vi "NF90 calibrator.vi"(9 "Ports":T1, 10 "channel index":i8, 11 "data server address":string="calcium") -> ()   [LabVIEW 2012]
doc: "Illustrates the simplest form of TCP data acquisition using a TCP data server.\n\n\nCreated by Monroe Weber-Shirk\nCornell University\nmw24@cornell.edu\nJanuary 2000"
uses:
  NF90 move.ctl
  Axis.ctl
  DAC apps/support/method.ctl
  DataServer/command cluster.ctl
  DataServer/command.ctl
  DAQ configuration/Sensor array.ctl
  DAQ configuration/channel identifier.ctl
  NF90 commands.ctl
  calibration/global scale array.vi
  DataServer/Server Stats.vi
panel:
  in  "Go to Start":bool
  in  "Save Data":bool
  in  "Save Calibration":bool
  in  "Calibrate":bool
  in  "Go Home":bool
  in  "Done":bool
  in  "Find Home":bool
  in  "Acceleration":u8=6 min=1 max=50 step=1
  in  "Speed":sgl=1.0 min=0 max=3 format="%.3f"
  out "sample time":dbl format="%.2f"
  out "Sample rate":dbl format="%.2f"
  out "Error":cluster{sgl[], dbl[]}[](graph)
  in  "polynomial order":i32=2 min=1 max=5 step=1
  out "Calibation data":cluster{sgl[], "Best Polynomial Fit":dbl[]}[](graph)
  in  "Number of locations":u8=5 min=2 step=1
  in  "Start position":sgl min=-1048575 max=1048575 format="%.2f"
  in  "delay after move":u32=1000
  in  "Final position":sgl=10.0 min=-1048575 max=1048575 format="%.2f"
  in  "data points to acquire":u32=1000 min=1
  in  "Scans per Sample":i32=1 min=1
  in  "Connection ID":refnum<k5>
  in  "method":T3={"sampling interval"=0.1, "samples to average"=1, "data interval"=0.0, "stream data"=FALSE, "file path"=refnum, "command"={"command"=enum."Idle", "start time (ms)"=0, "Channel Indices"=[], "Scans per Sample"=1}} {"command"."Scans per Sample" min=1; "data interval" format="%.2f"; "samples to average" min=1 step=1; "sampling interval" format="%.2f"}
  in  "move":T6={"axis"=enum."Z", "Increment"=0.0, "Speed"=1.0, "Acceleration"=1} {"Speed" min=0 format="%.3f"; "Acceleration" min=1 max=50 step=1; "Increment" format="%.3f"}
  in  "Home offset from limit switch":sgl min=-1048575 max=1048575 format="%.2f"
  out "Position":sgl(slide) min=0 max=6 step=-1 scale=0.0..1.0 scale format="%.2f"
  in  "serial port":refnum<visa-resource-name>="COM1"
  in  "stop":bool
  # "cm"
  # "cm/s"
  # "cm/s^2"
  # "cm"
  # "cm"
  # "Hz"
  # "s"
  # "ms"
  # "s"
  # "s"
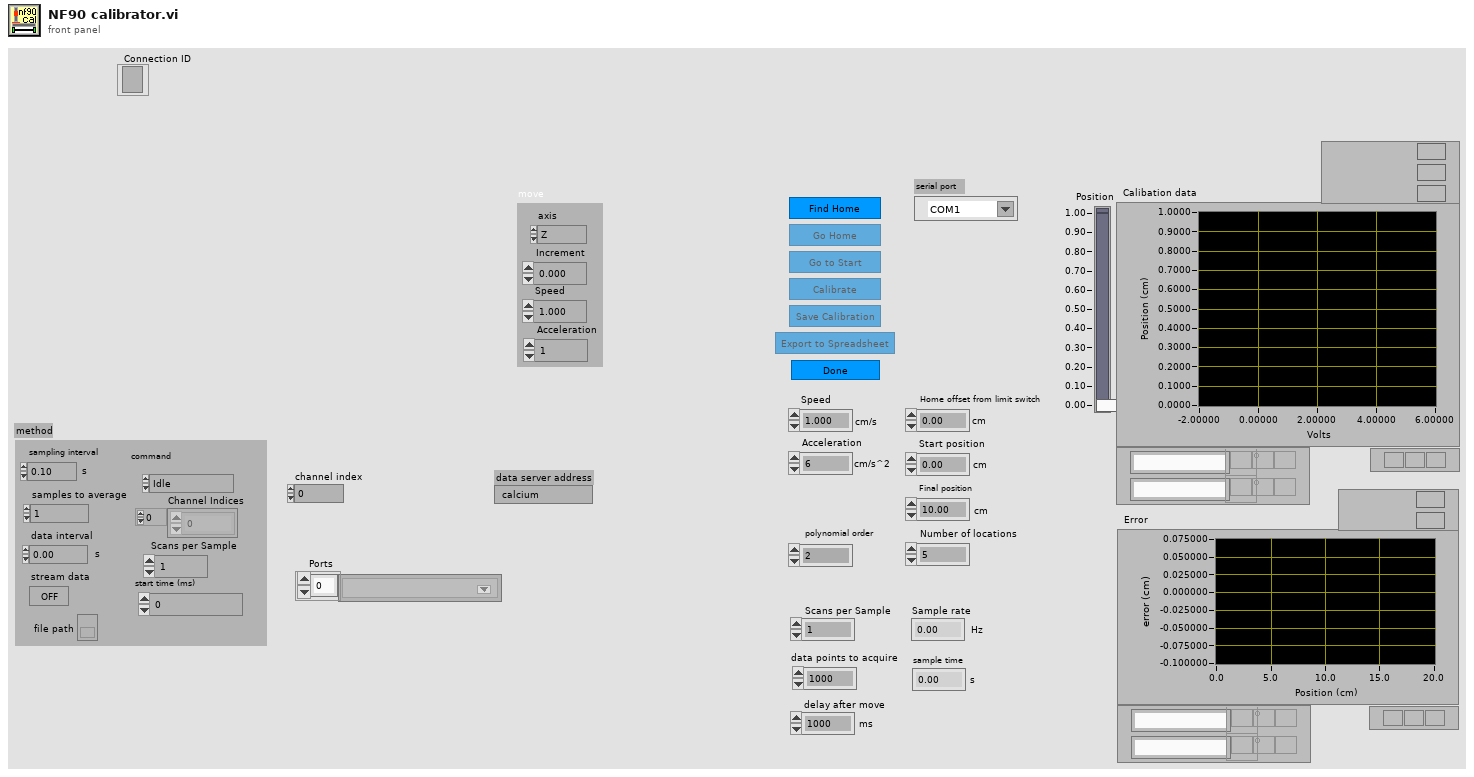
[diagram p1: front panel]
types:
  T1 = typedef "Sensor array.ctl" = T2[]
  T2 = typedef "channel identifier.ctl" = u16
  T3 = typedef "method.ctl" = cluster{"sampling interval":sgl, "samples to average":u32, "data interval":sgl, "stream data":bool, "file path":refnum<file>, "command":T4}
  T4 = typedef "command cluster.ctl" = cluster{"command":T5, "start time (ms)":u32, "Channel Indices":i32[], "Scans per Sample":i32}
  T5 = typedef "command.ctl" = enum16{"Idle", "Send Data", "Send 1 Scan", "Logoff"}
  T6 = typedef "NF90 move.ctl" = cluster{"axis":T7, "Increment":sgl, "Speed":sgl, "Acceleration":u8}
  T7 = typedef "Axis.ctl" = enum16{"X", "Y", "Z"}
  T8 = typedef "NF90 commands.ctl" = enum16{"Index", "Speed", "Acceleration", "Backlash", "Quit", "Run", "Null indexes", "Verify status", "Clear program", "Computer Control", "Go", "Put Controller on Hold", "Position"}
  T9 = typedef "calib array.ctl" = T10[]
  T10 = typedef "conversion.ctl" = cluster{"conversion matrix":sgl[][], "units":string, "name":string, "scale type":T11, "offset (volts)":dbl, "second channel":i8, "correspondence table":T12, "offset (physical units)":dbl, "pH scale":T13, "D.O.":T14}
  T11 = typedef "scale type.ctl" = enum16{"Volts", "Polynomial", "Correspondence Table", "pH", "Dissolved Oxygen", "Quadratic"}
  T12 = typedef "correspondence table.ctl" = cluster{"physical units":dbl, "volts":dbl}[]
  T13 = typedef "pH scale.ctl" = cluster{"Buffers":cluster{"Buffer":dbl, "Calibrated":bool, "V/T":dbl}[], "Temperature":dbl}
  T14 = typedef "DO scale.ctl" = cluster{"Temperature":dbl, "K":dbl, "barometric pressure":dbl}
  T15 = typedef "Server stats.ctl" = cluster{"scan rate":dbl, "# connections":i32, "channel settings":cluster{"Name":string, "upper input limits":sgl, "lower input limits":sgl, "Location":string}[]}
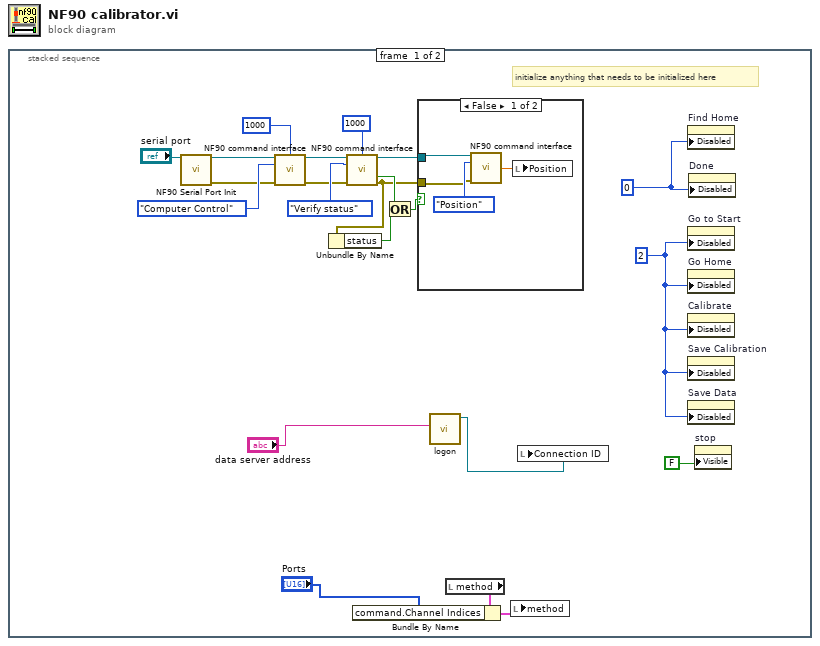
[diagram p0: block diagram]
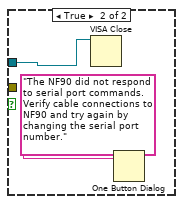
[diagram p2: hidden frame]
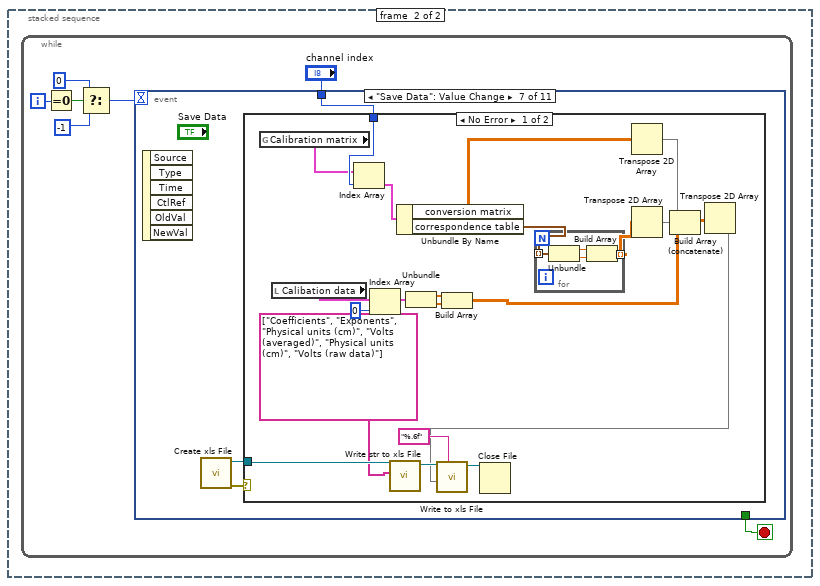
[diagram p3: hidden frame]
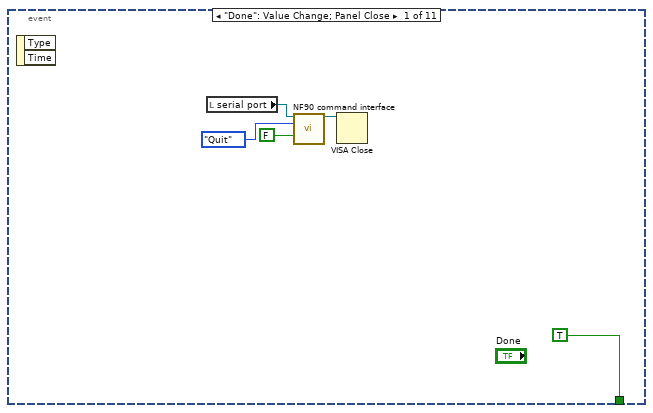
[diagram p4: hidden frame]
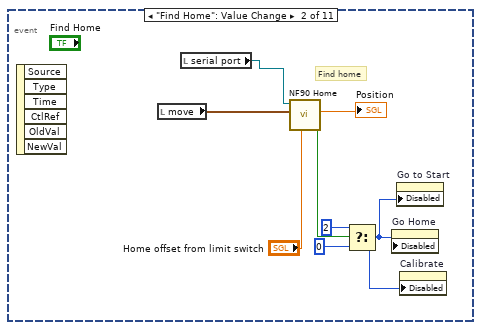
[diagram p5: hidden frame]
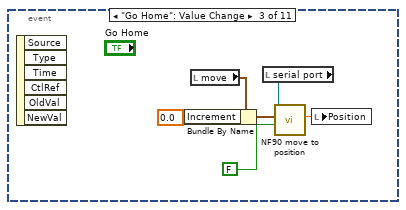
[diagram p6: hidden frame]
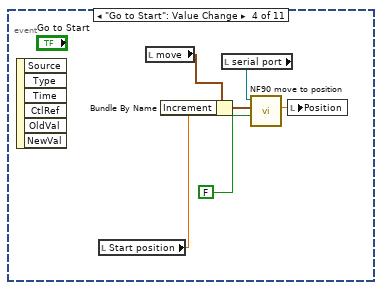
[diagram p7: hidden frame]
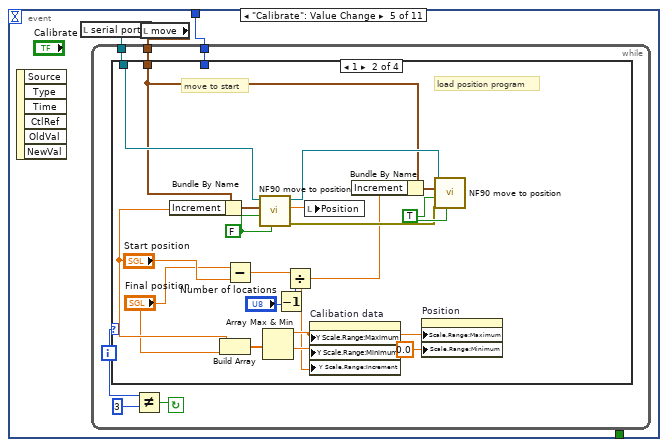
[diagram p8: hidden frame]
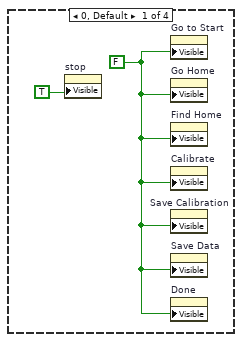
[diagram p9: hidden frame]
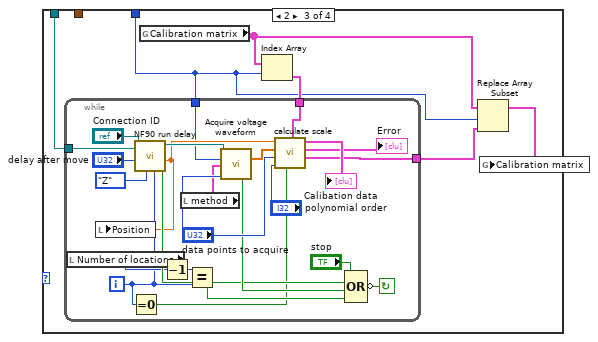
[diagram p10: hidden frame]
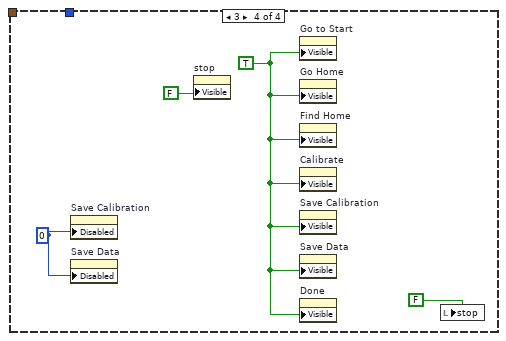
[diagram p11: hidden frame]
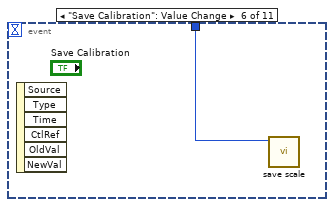
[diagram p12: hidden frame]
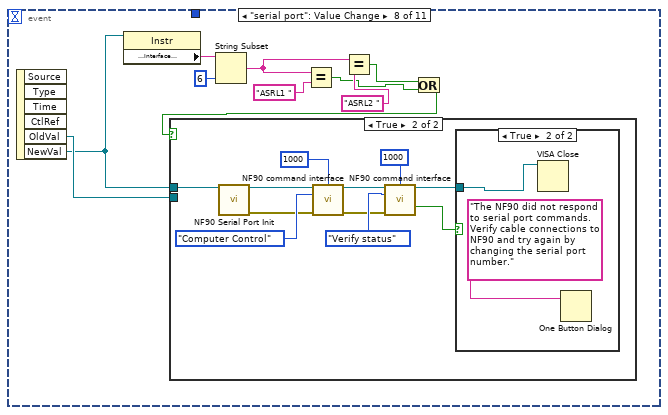
[diagram p14: hidden frame]
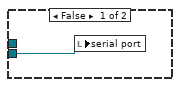
[diagram p15: hidden frame]
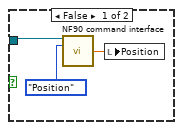
[diagram p16: hidden frame]
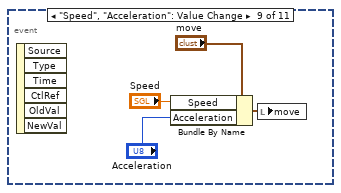
[diagram p17: hidden frame]
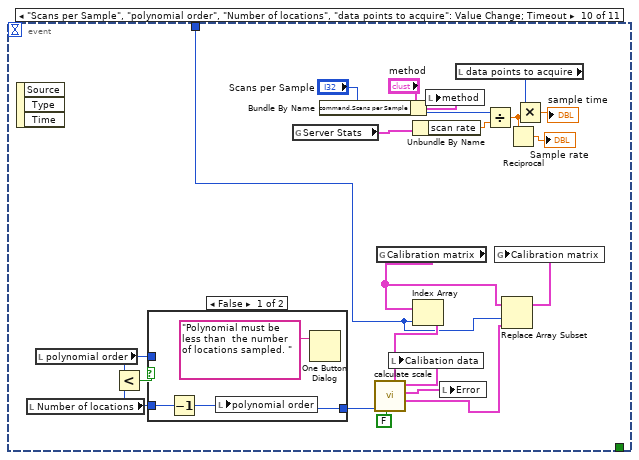
[diagram p18: hidden frame]
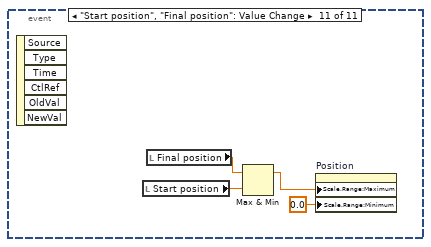
[diagram p20: hidden frame]
diagram:
  n1 = stacked-sequence {
    frame #0 {
      w10 = u8 2 ("Disabled")
      w9 = u8 0 ("Disabled")
      # "initialize anything that needs to be initialized here"
      n2 = call "NF90 Serial Port Init.vi"("port number"="serial port") -> ("port number"=w22:refnum<visa-resource-name>, "error out"=w7:errorcluster)  [unwired: 13 in]
      n3 = call "NF90 command interface.vi"("port number in"=w22, "time out (ms)"=u32 1000, "commands"=NF90_commands."Computer Control", "Error In"=w7) -> ("port number out"=w18:refnum<visa-resource-name>, "Error Out"=w6:errorcluster)  [unwired: 7 in, 3 out]
      n4 = call "NF90 command interface.vi"("port number in"=w18, "time out (ms)"=u32 1000, "commands"=NF90_commands."Verify status", "Error In"=w6) -> ("port number out"=w17:refnum<visa-resource-name>, "timed out"=w4:bool, "Error Out"=w2:errorcluster)  [unwired: 7 in, 2 out]
      n5 = Unbundle By Name(w2) -> ("status"=w5:bool)
      n6 = Or(x=w4, y=w5) -> (x .or. y?=w3:bool)
      n7 = case shown="False" w3 {
        tunnel: w17 -> [w24 w27]
        tunnel: w2 -> [w23 _]
        frame False {
          n8 = call "NF90 command interface.vi"("port number in"=w24, "commands"=NF90_commands."Position", "Error In"=w23) -> ("Position"=w25:sgl)  [unwired: 8 in, 4 out]
          n9 = local write "Position"(w25) -> ()
        }
        frame True {
          n10 = VISA Close(VISA resource name=w27) -> ()  [unwired: 1 in, 1 out]
          n11 = One Button Dialog(message="The NF90 did not respond to serial port commands. Verify cable connections to NF90 and try again by changing the serial port number.") -> ()  [unwired: 1 in, 1 out]
        }
      }
      n12 = call "logon.vi"("data server address in"="data server address") -> ("connection ID"=w11:refnum<k5>)  [unwired: 7 in, 3 out]
      n13 = local read "method"() -> (w14:T3)
      n14 = Bundle By Name(cluster=w14, "command.Channel Indices"="Ports") -> (w13:T3)
      n15 = local write "method"(w13) -> ()
      n16 = local write "Connection ID"(w11) -> ()
      n17 = property on="Find Home" class="Bool"("Disabled"=w9) -> ()  [unwired: 2 in, 2 out]
      n18 = property on="Go to Start" class="Bool"("Disabled"=w10) -> ()  [unwired: 2 in, 2 out]
      n19 = property on="Go Home" class="Bool"("Disabled"=w10) -> ()  [unwired: 2 in, 2 out]
      n20 = property on="Calibrate" class="Bool"("Disabled"=w10) -> ()  [unwired: 2 in, 2 out]
      n21 = property on="Save Calibration" class="Bool"("Disabled"=w10) -> ()  [unwired: 2 in, 2 out]
      n22 = property on="Save Data" class="Bool"("Disabled"=w10) -> ()  [unwired: 2 in, 2 out]
      n23 = property on="Done" class="Bool"("Disabled"=w9) -> ()  [unwired: 2 in, 2 out]
      n24 = property on="stop" class="Bool (strict)"("Visible"=FALSE) -> ()  [unwired: 2 in, 2 out]
    }
    frame #1 {
      n25 = while {
        i -> [w33]
        stop <- w34 stop-if-true
        n26 = Equal To 0?(x=w33) -> (x = 0?=w32:bool)
        n27 = Select(t=0, s=w32, f=-1) -> (s? t:f=w29:i32)
        n28 = event shown="[6] \"Save Data\": Value Change" {
          selector: _ -> [_ _ _ _ _ _ _ _ _ _ _]
          dyn-events: _ -> [_ _ _ _ _ _ _ _ _ _ _]
          timeout: w29 -> [_ _ _ _ _ _ _ _ _ _ _]
          tunnel: "channel index" -> [_ _ _ _ w63 w125 w126 _ _ w185 _]
          tunnel: [TRUE _ _ _ _ _ _ _ _ _ _] -> w34
          event "Done": Value Change; Panel Close {
            n29 = event-data() -> ()  [unwired: 1 in, 2 out]
            n30 = local read "serial port"() -> (w37:refnum<visa-resource-name>)
            n31 = call "NF90 command interface.vi"("port number in"=w37, "commands"=NF90_commands."Quit", "enable?"=FALSE) -> ("port number out"=w40:refnum<visa-resource-name>)  [unwired: 8 in, 4 out]
            n32 = VISA Close(VISA resource name=w40) -> ()  [unwired: 1 in, 1 out]
          }
          event "Find Home": Value Change {
            # "Find home"
            n33 = event-data() -> ()  [unwired: 1 in, 6 out]
            n34 = local read "move"() -> (w43:T6)
            n35 = local read "serial port"() -> (w42:refnum<visa-resource-name>)
            n36 = call "NF90 Home.vi"("Index offset from switch"="Home offset from limit switch", "move"=w43, "port number in"=w42) -> ("killed"=w46:bool, "position"=→"Position":dbl)  [unwired: 4 in, 2 out]
            n37 = Select(t=2, s=w46, f=0) -> (s? t:f=w41:i32)
            n38 = property on="Go Home" class="Bool"("Disabled"=w41) -> ()  [unwired: 2 in, 2 out]
            n39 = property on="Go to Start" class="Bool"("Disabled"=w41) -> ()  [unwired: 2 in, 2 out]
            n40 = property on="Calibrate" class="Bool"("Disabled"=w41) -> ()  [unwired: 2 in, 2 out]
          }
          event "Go Home": Value Change {
            n41 = event-data() -> ()  [unwired: 1 in, 6 out]
            n42 = local read "move"() -> (w49:T6)
            n43 = Bundle By Name(cluster=w49, "Increment"=sgl 0.0 ("Bundle Element")) -> (w51:T6)
            n44 = local read "serial port"() -> (w50:refnum<visa-resource-name>)
            n45 = call "NF90 move to position.vi"("move type (abs = False)"=FALSE ("move type (abs = true)"), "move"=w51, "port number in"=w50) -> ("Position out"=w54:sgl)  [unwired: 4 in, 3 out]
            n46 = local write "Position"(w54) -> ()
          }
          event "Go to Start": Value Change {
            n47 = event-data() -> ()  [unwired: 1 in, 6 out]
            n48 = local read "Start position"() -> (w60:sgl)
            n49 = local read "move"() -> (w55:T6)
            n50 = Bundle By Name(cluster=w55, "Increment"=w60) -> (w57:T6)
            n51 = local read "serial port"() -> (w56:refnum<visa-resource-name>)
            n52 = call "NF90 move to position.vi"("move type (abs = False)"=FALSE ("move type (abs = true)"), "move"=w57, "port number in"=w56) -> ("Position out"=w59:sgl)  [unwired: 4 in, 3 out]
            n53 = local write "Position"(w59) -> ()
          }
          event "Calibrate": Value Change {
            n54 = event-data() -> ()  [unwired: 1 in, 6 out]
            n55 = local read "serial port"() -> (w62:refnum<visa-resource-name>)
            n56 = local read "move"() -> (w61:T6)
            n57 = while {
              tunnel: w62 -> [w67]
              tunnel: w61 -> [w68]
              tunnel: w63 -> [w64]
              i -> [w69]
              stop <- w65 continue-if-true
              n58 = case shown="1" w69 {
                tunnel: w68 -> [_ w83 _ _]
                tunnel: w67 -> [_ w89 w96 _]
                tunnel: w64 -> [_ _ w91 _]
                frame 0, Default {
                  w71 = FALSE ("Visible")
                  n59 = property on="stop" class="Bool (strict)"("Visible"=TRUE) -> ()  [unwired: 2 in, 2 out]
                  n60 = property on="Go to Start" class="Bool"("Visible"=w71) -> ()  [unwired: 2 in, 2 out]
                  n61 = property on="Go Home" class="Bool"("Visible"=w71) -> ()  [unwired: 2 in, 2 out]
                  n62 = property on="Find Home" class="Bool"("Visible"=w71) -> ()  [unwired: 2 in, 2 out]
                  n63 = property on="Calibrate" class="Bool"("Visible"=w71) -> ()  [unwired: 2 in, 2 out]
                  n64 = property on="Save Calibration" class="Bool"("Visible"=w71) -> ()  [unwired: 2 in, 2 out]
                  n65 = property on="Save Data" class="Bool"("Visible"=w71) -> ()  [unwired: 2 in, 2 out]
                  n66 = property on="Done" class="Bool"("Visible"=w71) -> ()  [unwired: 2 in, 2 out]
                }
                frame 1 {
                  w82 = FALSE ("move type (abs = true)")
                  w81 = TRUE ("move type (abs = False)")
                  # "move to start"
                  # "load position program"
                  n67 = Bundle By Name(cluster=w83, "Increment"="Start position") -> (w90:T6)
                  n68 = Build Array("Start position", "Final position") -> (w76:sgl[])
                  n69 = Subtract(x="Final position", y="Start position") -> (x-y=w86:sgl)
                  n70 = call "NF90 move to position.vi"("program (Run=False)"=w82, "move type (abs = False)"=w82, "move"=w90, "port number in"=w89) -> ("Error Out"=w80:errorcluster, "Position out"=w79:sgl, "port number out"=w88:refnum<visa-resource-name>)  [unwired: 3 in, 1 out]
                  n71 = Array Max & Min(array=w76) -> (max value=w75:sgl, min value=w74:sgl)  [unwired: 2 out]
                  n72 = Decrement(x="Number of locations") -> (x-1=w85:u8)
                  n73 = Divide(x=w86, y=w85) -> (x/y=w73:sgl)
                  n74 = local write "Position"(w79) -> ()
                  n75 = property on="Calibation data" class="XYGraph (strict)"("Y Scale.Range:Maximum"=w75, "Y Scale.Range:Minimum"=w74, "Y Scale.Range:Increment"=w73) -> ()  [unwired: 2 in, 2 out]
                  n76 = Bundle By Name(cluster=w83, "Increment"=w73) -> (w84:T6)
                  n77 = property on="Position" class="Slide (strict)"("Scale.Range:Maximum"=w75, "Scale.Range:Minimum"=0.0) -> ()  [unwired: 2 in, 2 out]
                  n78 = call "NF90 move to position.vi"("program (Run=False)"=w81, "Error In"=w80, "move type (abs = False)"=w81, "move"=w84, "port number in"=w88) -> ()  [unwired: 2 in, 4 out]
                }
                frame 2 {
                  n79 = global read "global scale array.vi" "Calibration matrix"() -> (w94:T9)
                  n80 = Index Array(array=w94, index=w91) -> (element=w95:T10)
                  n81 = while {
                    tunnel: [w105] -> w93
                    tunnel: w96 -> [w120]
                    tunnel: w91 -> [w98]
                    tunnel: w95 -> [w97]
                    i -> [w100]
                    stop <- w115 continue-if-true
                    n82 = local read "Number of locations"() -> (w111:u8)
                    n83 = Equal To 0?(x=w100) -> (x = 0?=w99:bool)
                    n84 = call "NF90 run delay.vi"("i"=w100, "axis"=Axis."Z", "delay (ms)"="delay after move", "port number"=w120, "Connection ID"="Connection ID") -> ("Position"=w107:sgl, "killed"=w113:bool, "Connection ID out"=w117:refnum<k5>)  [unwired: 3 in, 1 out]
                    n85 = local write "Position"(w107) -> ()
                    n86 = Decrement(x=w111) -> (x-1=w104:u8)
                    n87 = local read "method"() -> (w101:T3)
                    n88 = Equal?(x=w104, y=w100) -> (x = y?=w110:bool)
                    n89 = call "Acquire voltage waveform.vi"("Connection ID"=w117, "channel index"=w98, "method"=w101, "data points to acquire"="data points to acquire") -> ("channel data array"=w108:sgl[], "canceled"=w114:bool)  [unwired: 6 in, 4 out]
                    n90 = call "calculate scale.vi"("Scaling in"=w97, "reset"=w99, "polynomial order"="polynomial order", "data points to acquire"="data points to acquire", "volts array"=w108, "Position"=w107) -> ("Scaling out"=w105:T10, "error graph"=→"Error":cluster{"X array":sgl[], "Y array":dbl[]}[], "Output Graph"=→"Calibation data":cluster{"X array":sgl[], "Y array":dbl[]}[])  [unwired: 2 in]
                    n91 = Compound Arithmetic op=OR("stop", w113, w114, w110) -> (invert w115:bool)
                  }
                  n92 = Replace Array Subset(array=w94, new element=w93, index=w91) -> (w92:T9)
                  n93 = global write "global scale array.vi" "Calibration matrix"(w92) -> ()
                }
                frame 3 {
                  w123 = TRUE ("Visible")
                  w121 = u8 0 ("Disabled")
                  n94 = property on="Save Calibration" class="Bool"("Disabled"=w121) -> ()  [unwired: 2 in, 2 out]
                  n95 = property on="Save Data" class="Bool"("Disabled"=w121) -> ()  [unwired: 2 in, 2 out]
                  n96 = property on="stop" class="Bool (strict)"("Visible"=FALSE) -> ()  [unwired: 2 in, 2 out]
                  n97 = property on="Go to Start" class="Bool"("Visible"=w123) -> ()  [unwired: 2 in, 2 out]
                  n98 = property on="Go Home" class="Bool"("Visible"=w123) -> ()  [unwired: 2 in, 2 out]
                  n99 = property on="Find Home" class="Bool"("Visible"=w123) -> ()  [unwired: 2 in, 2 out]
                  n100 = property on="Calibrate" class="Bool"("Visible"=w123) -> ()  [unwired: 2 in, 2 out]
                  n101 = property on="Save Calibration" class="Bool"("Visible"=w123) -> ()  [unwired: 2 in, 2 out]
                  n102 = property on="Save Data" class="Bool"("Visible"=w123) -> ()  [unwired: 2 in, 2 out]
                  n103 = property on="Done" class="Bool"("Visible"=w123) -> ()  [unwired: 2 in, 2 out]
                  n104 = local write "stop"(FALSE ("Visible")) -> ()
                }
              }
              n105 = Not Equal?(x=w69, y=3) -> (x != y?=w65:bool)
            }
          }
          event "Save Calibration": Value Change {
            n106 = event-data() -> ()  [unwired: 1 in, 6 out]
            n107 = call "save scale.vi"("Index"=w125) -> ()  [unwired: 6 in, 1 out]
          }
          event "Save Data": Value Change {
            n108 = event-data() -> ()  [unwired: 1 in, 6 out]
            n109 = call "Create xls File.vi"() -> ("error out"=w128:errorcluster, "refnum"=w127:refnum<file>)  [unwired: 4 in, 2 out]
            n110 = case shown="No Error" w128 {
              tunnel: w127 -> [w133 _]
              tunnel: w126 -> [w132 _]
              frame No Error {
                n111 = global read "global scale array.vi" "Calibration matrix"() -> (w131:T9)
                n112 = local read "Calibation data"() -> (w137:cluster{sgl[], "Best Polynomial Fit":dbl[]}[])
                n113 = Index Array(array=w131, index=w132) -> (element=w130:T10)
                n114 = Index Array(array=w137, index=0 ("Index")) -> (element=w136:cluster{sgl[], "Best Polynomial Fit":dbl[]})
                n115 = call "Write str to xls File.vi"("1D data"=string[] ["Coefficients", "Exponents", "Physical units (cm)", "Volts (averaged)", "Physical units (cm)", "Volts (raw data)"], "refnum"=w133) -> ("dup refnum"=w149:refnum<file>)  [unwired: 8 in, 1 out]
                n116 = Unbundle By Name(w130) -> ("conversion matrix"=w144:sgl[][], "correspondence table"=w147:T12)
                n117 = Unbundle(w136) -> (w139:sgl[], "Best Polynomial Fit"=w138:dbl[])
                n118 = Build Array(w139, w138) -> (w134:dbl[][])
                n119 = for {
                  tunnel: w147 -> [w153] mode=indexing
                  tunnel: [w150] -> w146 mode=indexing
                  n120 = Unbundle(w153) -> ("physical units"=w152:dbl, "volts"=w151:dbl)
                  n121 = Build Array(w152, w151) -> (w150:dbl[])
                }
                n122 = Transpose 2D Array(2D array=w144) -> (transposed array=w142:sgl[][])
                n123 = Transpose 2D Array(2D array=w146) -> (transposed array=w141:dbl[][])
                n124 = Build Array (concatenate)(w142, w141, w134) -> (w145:dbl[][])
                n125 = Transpose 2D Array(2D array=w145) -> (transposed array=w140:dbl[][])
                n126 = call "Write to xls File.vi"("format (%.3f)"="%.6f", "2D data"=w140, "refnum"=w149) -> ("dup refnum"=w148:refnum<file>)  [unwired: 7 in, 1 out]
                n127 = Close File(refnum=w148) -> ()  [unwired: 1 in, 2 out]
              }
              frame Error {
              }
            }
          }
          event "serial port": Value Change {
            n128 = event-data() -> ("OldVal"=w162:refnum<visa-resource-name>, "NewVal"=w154:refnum<visa-resource-name>)  [unwired: 1 in, 4 out]
            n129 = property class="Instr"(reference=w154) -> ("Interface Information:Interface Description"=w157:string)  [unwired: 1 in, 2 out]
            n130 = String Subset(string=w157, length (rest)=6 ("length (rest)")) -> (substring=w156:string)  [unwired: 1 in]
            n131 = Equal?(x=w156, y="ASRL1 ") -> (x = y?=w159:bool)
            n132 = Equal?(x=w156, y="ASRL2 ") -> (x = y?=w160:bool)
            n133 = Or(x=w160, y=w159) -> (x .or. y?=w158:bool)
            n134 = case shown="True" w158 {
              tunnel: w154 -> [_ w165]
              tunnel: w162 -> [w164 _]
              frame False {
                n135 = local write "serial port"(w164) -> ()
              }
              frame True {
                n136 = call "NF90 Serial Port Init.vi"("port number"=w165) -> ("port number"=w175:refnum<visa-resource-name>, "error out"=w167:errorcluster)  [unwired: 13 in]
                n137 = call "NF90 command interface.vi"("port number in"=w175, "time out (ms)"=u32 1000, "commands"=NF90_commands."Computer Control", "Error In"=w167) -> ("port number out"=w172:refnum<visa-resource-name>, "Error Out"=w166:errorcluster)  [unwired: 7 in, 3 out]
                n138 = call "NF90 command interface.vi"("port number in"=w172, "time out (ms)"=u32 1000, "commands"=NF90_commands."Verify status", "Error In"=w166) -> ("port number out"=w171:refnum<visa-resource-name>, "timed out"=w168:bool)  [unwired: 7 in, 3 out]
                n139 = case shown="True" w168 {
                  tunnel: w171 -> [w176 w179]
                  frame False {
                    n140 = call "NF90 command interface.vi"("port number in"=w176, "commands"=NF90_commands."Position") -> ("Position"=w177:sgl)  [unwired: 9 in, 4 out]
                    n141 = local write "Position"(w177) -> ()
                  }
                  frame True {
                    n142 = VISA Close(VISA resource name=w179) -> ()  [unwired: 1 in, 1 out]
                    n143 = One Button Dialog(message="The NF90 did not respond to serial port commands. Verify cable connections to NF90 and try again by changing the serial port number.") -> ()  [unwired: 1 in, 1 out]
                  }
                }
              }
            }
          }
          event "Speed", "Acceleration": Value Change {
            n144 = event-data() -> ()  [unwired: 1 in, 6 out]
            n145 = Bundle By Name(cluster="move", "Speed"="Speed", "Acceleration"="Acceleration") -> (w181:T6)
            n146 = local write "move"(w181) -> ()
          }
          event "Scans per Sample", "polynomial order", "Number of locations", "data points to acquire": Value Change; Timeout {
            n147 = event-data() -> ()  [unwired: 1 in, 3 out]
            n148 = local read "Number of locations"() -> (w188:u8)
            n149 = local read "polynomial order"() -> (w186:i32)
            n150 = Less?(x=w186, y=w188) -> (x < y?=w187:bool)
            n151 = case shown="False" w187 {
              tunnel: w188 -> [w208 _]
              tunnel: [w206 w209] -> w189
              tunnel: w186 -> [_ w209]
              frame False {
                n152 = Decrement(x=w208) -> (x-1=w206:u8)
                n153 = local write "polynomial order"(w206) -> ()
                n154 = One Button Dialog(message="Polynomial must be less than  the number of locations sampled. ") -> ()  [unwired: 1 in, 1 out]
              }
              frame True {
              }
            }
            n155 = global read "Server Stats.vi" "Server Stats"() -> (w205:T15)
            n156 = Bundle By Name(cluster="method", "command.Scans per Sample"="Scans per Sample") -> (w200:T3)
            n157 = global read "global scale array.vi" "Calibration matrix"() -> (w193:T9)
            n158 = Unbundle By Name(w205) -> ("scan rate"=w197:dbl)
            n159 = Index Array(array=w193, index=w185) -> (element=w195:T10)
            n160 = call "calculate scale.vi"("Scaling in"=w195, "reset"=FALSE, "polynomial order"=w189) -> ("Scaling out"=w196:T10, "error graph"=w191:cluster{"X array":sgl[], "Y array":dbl[]}[], "Output Graph"=w190:cluster{"X array":sgl[], "Y array":dbl[]}[])  [unwired: 5 in]
            n161 = local write "Calibation data"(w190) -> ()
            n162 = local write "method"(w200) -> ()
            n163 = local write "Error"(w191) -> ()
            n164 = local read "data points to acquire"() -> (w201:u32)
            n165 = Divide(x="Scans per Sample", y=w197) -> (x/y=w203:dbl)
            n166 = Replace Array Subset(array=w193, new element=w196, index=w185) -> (w194:T9)
            n167 = global write "global scale array.vi" "Calibration matrix"(w194) -> ()
            n168 = Reciprocal(x=w203) -> (1/x=→"Sample rate":dbl)
            n169 = Multiply(x=w201, y=w203) -> (x*y=→"sample time":dbl)
          }
          event "Start position", "Final position": Value Change {
            n170 = event-data() -> ()  [unwired: 1 in, 6 out]
            n171 = local read "Start position"() -> (w212:sgl)
            n172 = local read "Final position"() -> (w213:sgl)
            n173 = Max & Min(x=w213, y=w212) -> (max(x,y)=w211:sgl)  [unwired: 1 out]
            n174 = property on="Position" class="Slide (strict)"("Scale.Range:Maximum"=w211, "Scale.Range:Minimum"=0.0) -> ()  [unwired: 2 in, 2 out]
          }
        }
      }
    }
  }
